vi "Check Direction.vi"(8 "error in (no error)":errorcluster, 11 "Controller Data Cluster":T2) -> (0 "error out":errorcluster, 3 "Direction":T1)   [LabVIEW 2017]
uses:
  Controller Data Cluster.ctl
  User Console/UI Data Cluster.ctl
  Timed Action.ctl
  Current Direction.ctl
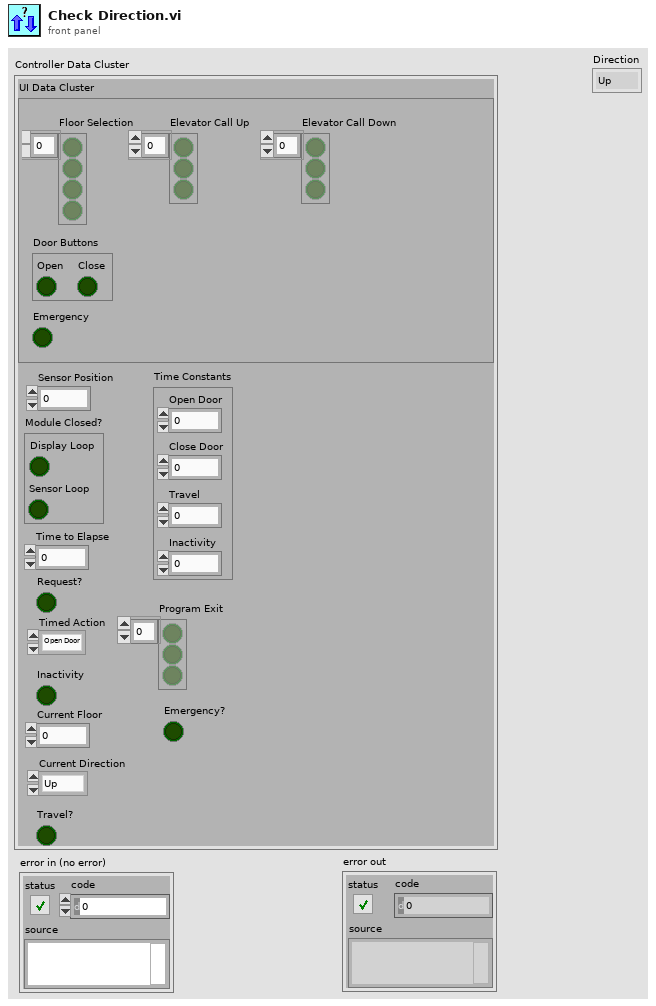
[diagram p1: front panel]
types:
  T1 = typedef "Current Direction.ctl" = enum16{"Up", "Down", "Idle"}
  T2 = typedef "Controller Data Cluster.ctl" = cluster{"UI Data Cluster":T3, "Sensor Position":u32, "Module Closed?":cluster{"Display Loop":bool, "Sensor Loop ":bool}, "Time to Elapse":u32, "Request?":bool, "Timed Action":T4, "Time Constants":cluster{"Open Door":dbl, "Close Door":dbl, "Travel":dbl, "Inactivity":dbl}, "Inactivity":bool, "Current Floor":u32, "Current Direction":T1, "Travel?":bool, "Program Exit":bool[], "Emergency?":bool}
  T3 = typedef "UI Data Cluster.ctl" = cluster{"Floor Selection":bool[], "Elevator Call Up":bool[], "Elevator Call Down":bool[], "Door Buttons":cluster{"Open":bool, "Close":bool}, "Emergency":bool}
  T4 = typedef "Timed Action.ctl" = enum16{"Open Door", "Close Door", "Travel", "Inactivity"}
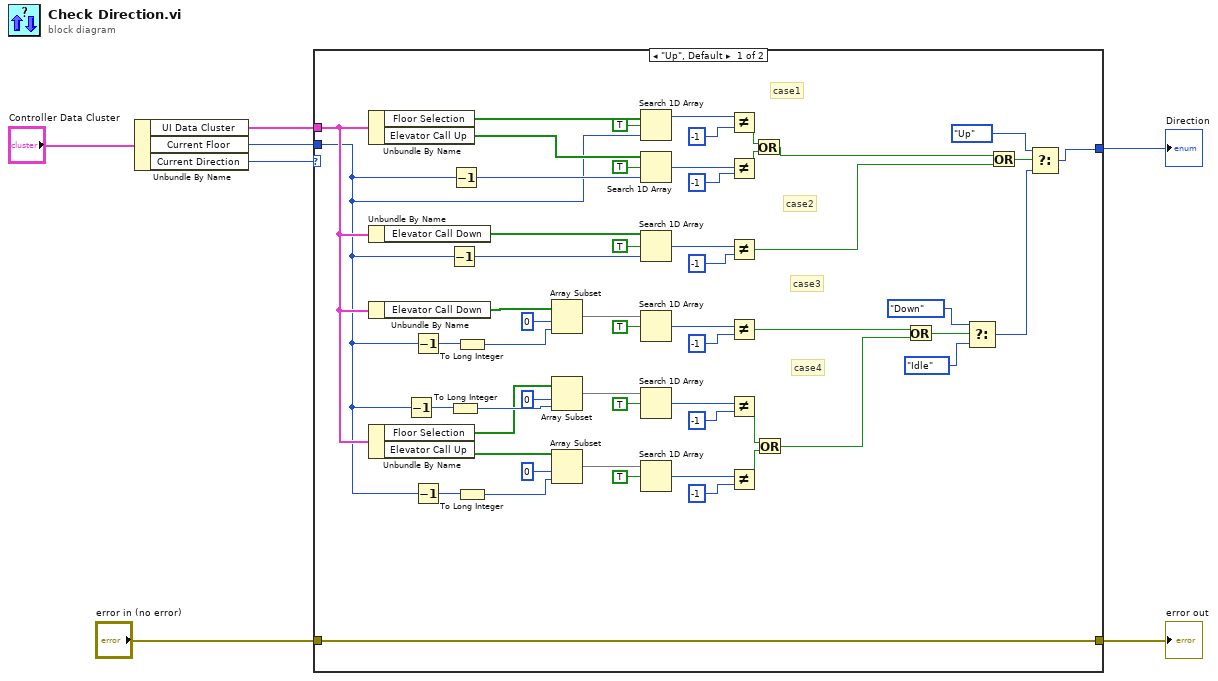
[diagram p0: block diagram]
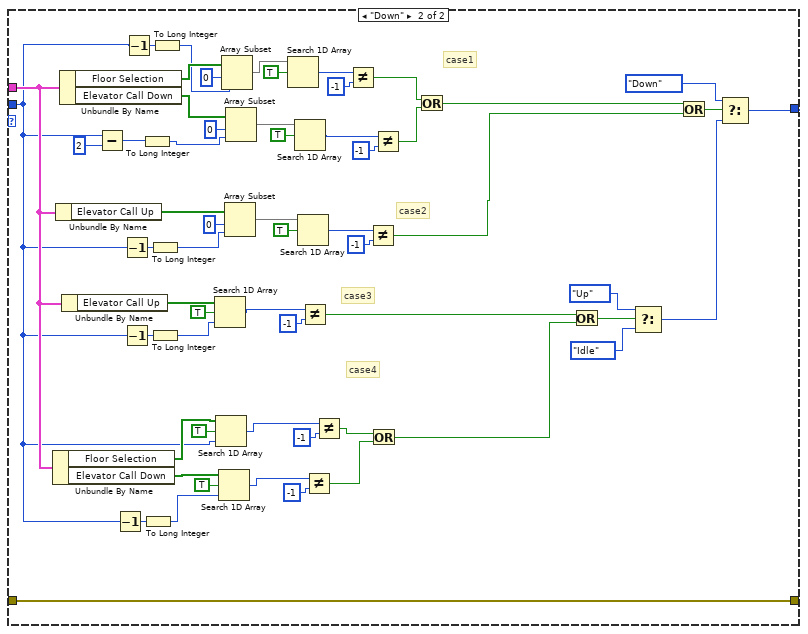
[diagram p2: hidden frame]
diagram:
  n1 = Unbundle By Name("Controller Data Cluster") -> ("UI Data Cluster"=w5:T3, "Current Floor"=w6:u32, "Current Direction"=w7:T1)
  n2 = case shown="\"Up\", Default" w7 {
    tunnel: w6 -> [w9 w80]
    tunnel: w5 -> [w21 w90]
    tunnel: [w10 w65] -> w3
    tunnel: [w8 w64] -> w2
    tunnel: "error in (no error)" -> [w8 w64]
    frame "Up", Default {
      # "case4"
      # "case3"
      # "case2"
      # "case1"
      n3 = Unbundle By Name(w21) -> ("Floor Selection"=w63:bool[], "Elevator Call Up"=w60:bool[])
      n4 = Unbundle By Name(w21) -> ("Elevator Call Down"=w53:bool[])
      n5 = Unbundle By Name(w21) -> ("Elevator Call Down"=w48:bool[])
      n6 = Unbundle By Name(w21) -> ("Floor Selection"=w29:bool[], "Elevator Call Up"=w33:bool[])
      n7 = Decrement(x=w9) -> (x-1=w32:u32)
      n8 = Decrement(x=w9) -> (x-1=w46:u32)
      n9 = Decrement(x=w9) -> (x-1=w35:u32)
      n10 = Decrement(x=w9) -> (x-1=w51:u32)
      n11 = To Long Integer(number=w32) -> (32bit integer=w30:i32)
      n12 = Decrement(x=w9) -> (x-1=w22:u32)
      n13 = To Long Integer(number=w46) -> (32bit integer=w45:i32)
      n14 = To Long Integer(number=w35) -> (32bit integer=w36:i32)
      n15 = Array Subset(array=w48, index=0, length=w45) -> (w43:bool[])
      n16 = Array Subset(array=w29, index=0, length=w30) -> (w27:bool[])
      n17 = Array Subset(array=w33, index=0, length=w36) -> (w38:bool[])
      n18 = Search 1D Array(1D array=w63, element=TRUE, start index (0)=w9) -> (index of element=w59:i32)
      n19 = Search 1D Array(1D array=w60, element=TRUE, start index (0)=w22) -> (index of element=w56:i32)
      n20 = Search 1D Array(1D array=w53, element=TRUE, start index (0)=w51) -> (index of element=w49:i32)
      n21 = Search 1D Array(1D array=w43, element=TRUE) -> (index of element=w41:i32)  [unwired: 1 in]
      n22 = Search 1D Array(1D array=w27, element=TRUE) -> (index of element=w25:i32)  [unwired: 1 in]
      n23 = Search 1D Array(1D array=w38, element=TRUE) -> (index of element=w40:i32)  [unwired: 1 in]
      n24 = Not Equal?(x=w59, y=-1) -> (x != y?=w55:bool)
      n25 = Not Equal?(x=w56, y=-1) -> (x != y?=w54:bool)
      n26 = Not Equal?(x=w49, y=-1) -> (x != y?=w17:bool)
      n27 = Not Equal?(x=w41, y=-1) -> (x != y?=w13:bool)
      n28 = Not Equal?(x=w25, y=-1) -> (x != y?=w24:bool)
      n29 = Not Equal?(x=w40, y=-1) -> (x != y?=w23:bool)
      n30 = Or(x=w55, y=w54) -> (x .or. y?=w18:bool)
      n31 = Or(x=w24, y=w23) -> (x .or. y?=w12:bool)
      n32 = Or(x=w13, y=w12) -> (x .or. y?=w16:bool)
      n33 = Select(t=Current_Direction."Down" ("Current Direction"), s=w16, f=Current_Direction."Idle") -> (s? t:f=w11:T1)
      n34 = Or(x=w18, y=w17) -> (x .or. y?=w20:bool)
      n35 = Select(t=Current_Direction."Up" ("Current Direction"), s=w20, f=w11) -> (s? t:f=w10:T1)
    }
    frame "Down" {
      # "case4"
      # "case3"
      # "case2"
      # "case1"
      n36 = Unbundle By Name(w90) -> ("Floor Selection"=w82:bool[], "Elevator Call Down"=w88:bool[])
      n37 = Unbundle By Name(w90) -> ("Elevator Call Up"=w103:bool[])
      n38 = Unbundle By Name(w90) -> ("Floor Selection"=w122:bool[], "Elevator Call Down"=w115:bool[])
      n39 = Unbundle By Name(w90) -> ("Elevator Call Up"=w95:bool[])
      n40 = Subtract(x=w80, y=u32 2) -> (x-y=w106:u32)
      n41 = Decrement(x=w80) -> (x-1=w89:u32)
      n42 = Decrement(x=w80) -> (x-1=w101:u32)
      n43 = Decrement(x=w80) -> (x-1=w93:u32)
      n44 = Decrement(x=w80) -> (x-1=w121:u32)
      n45 = To Long Integer(number=w106) -> (32bit integer=w105:i32)
      n46 = To Long Integer(number=w89) -> (32bit integer=w87:i32)
      n47 = To Long Integer(number=w101) -> (32bit integer=w100:i32)
      n48 = To Long Integer(number=w93) -> (32bit integer=w83:i32)
      n49 = To Long Integer(number=w121) -> (32bit integer=w114:i32)
      n50 = Search 1D Array(1D array=w95, element=TRUE, start index (0)=w83) -> (index of element=w91:i32)
      n51 = Search 1D Array(1D array=w82, element=TRUE, start index (0)=w80) -> (index of element=w78:i32)
      n52 = Search 1D Array(1D array=w88, element=TRUE, start index (0)=w87) -> (index of element=w84:i32)
      n53 = Array Subset(array=w122, index=0, length=w114) -> (w119:bool[])
      n54 = Array Subset(array=w103, index=0, length=w100) -> (w98:bool[])
      n55 = Array Subset(array=w115, index=0, length=w105) -> (w112:bool[])
      n56 = Search 1D Array(1D array=w119, element=TRUE) -> (index of element=w117:i32)  [unwired: 1 in]
      n57 = Search 1D Array(1D array=w112, element=TRUE) -> (index of element=w110:i32)  [unwired: 1 in]
      n58 = Search 1D Array(1D array=w98, element=TRUE) -> (index of element=w96:i32)  [unwired: 1 in]
      n59 = Not Equal?(x=w91, y=-1) -> (x != y?=w71:bool)
      n60 = Not Equal?(x=w84, y=-1) -> (x != y?=w77:bool)
      n61 = Not Equal?(x=w78, y=-1) -> (x != y?=w76:bool)
      n62 = Not Equal?(x=w117, y=-1) -> (x != y?=w109:bool)
      n63 = Not Equal?(x=w96, y=-1) -> (x != y?=w74:bool)
      n64 = Or(x=w76, y=w77) -> (x .or. y?=w70:bool)
      n65 = Not Equal?(x=w110, y=-1) -> (x != y?=w108:bool)
      n66 = Or(x=w109, y=w108) -> (x .or. y?=w75:bool)
      n67 = Or(x=w71, y=w70) -> (x .or. y?=w69:bool)
      n68 = Select(t=Current_Direction."Up" ("Current Direction"), s=w69, f=Current_Direction."Idle") -> (s? t:f=w66:T1)
      n69 = Or(x=w75, y=w74) -> (x .or. y?=w73:bool)
      n70 = Select(t=Current_Direction."Down" ("Current Direction"), s=w73, f=w66) -> (s? t:f=w65:T1)
    }
  }
  "Direction" <- w3
  "error out" <- w2
